vi "Roasting_Process (SubVI).vi"(10 "Array in":string[](array[string]), 11 "Digital in":refnum<vi>) -> (1 "Boolean":bool, 2 "Array out":string[](array[string]), 3 "empty?":bool)   [LabVIEW 2019]
uses:
  <vilib>/numeric/Random Number (Range) DBL.vi
  559fc5d8-92b6-4e94-9428-5fdf66a92b5f.vi
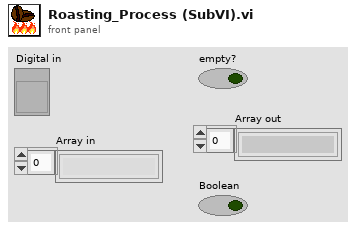
[diagram p1: front panel]
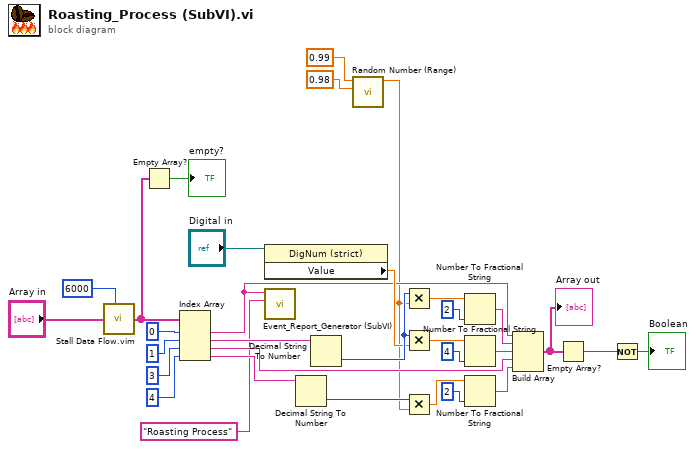
[diagram p0: block diagram]
diagram:
  n1 = call "Stall Data Flow.vim"("value in"="Array in", "milliseconds to wait"=u32 6000) -> ("value out"=w15:string[])  [unwired: 1 out]
  n2 = Empty Array?(array=w15) -> (empty?=→"empty?":bool)
  n3 = Index Array(array=w15, index #1=0 ("index"), index #2=1 ("index"), index #3=3 ("index"), index #4=4 ("index")) -> (element #1=w4:string, element #2=w13:string, element #3=w25:string, element #4=w26:string)
  n4 = property class="DigNum (strict)"(reference="Digital in") -> ("Value"=w23:dbl)  [unwired: 1 in, 2 out]
  n5 = call "Event_Report_Generator (SubVI).vi"("Process Name"="Roasting Process", "Booking ID"=w4) -> ()  [unwired: 10 in]
  n6 = Decimal String To Number(string=w26) -> (number=w27:i32)  [unwired: 2 in, 1 out]
  n7 = Decimal String To Number(string=w13) -> (number=w24:i32)  [unwired: 2 in, 1 out]
  n8 = call-poly <vilib>:"Random Number (Range).vi"("lower bound (0)"=0.98, "upper bound (100)"=0.99) -> ("number"=w1:dbl)  [unwired: 9 in]
  n9 = Multiply(x=w24, y=w1) -> (x*y=w19:dbl)
  n10 = Multiply(x=w24, y=w23) -> (x*y=w20:dbl)
  n11 = Multiply(x=w27, y=w1) -> (x*y=w29:dbl)
  n12 = Number To Fractional String(number=w19, precision (6)=i16 2) -> (F-format string=w22:string)  [unwired: 2 in]
  n13 = Number To Fractional String(number=w20, precision (6)=i16 4) -> (F-format string=w21:string)  [unwired: 2 in]
  n14 = Number To Fractional String(number=w29, precision (6)=i16 2) -> (F-format string=w30:string)  [unwired: 2 in]
  n15 = Build Array(w4, w22, w21, w25, w30) -> (w3:string[])
  "Array out" <- w3
  n16 = Empty Array?(array=w3) -> (empty?=w31:bool)
  n17 = Not(x=w31) -> (.not. x?=→"Boolean":bool)
